vi "populate ring from channel.vi"(7 "instance id":string, 8 "error in":errorcluster, 9 "channel":refnum<class "TBM channel.lvclass">, 10 "ring":refnum<vi>, 11 "engine configuration in":refnum<class "engine configuration.lvclass">) -> (0 "error out":errorcluster, 2 "mapped":bool, 3 "engine configuration out":refnum<class "engine configuration.lvclass">)   [LabVIEW 2013, in "configuration tests.lvlib" / "TEST EDITOR.lvclass"]
uses:
  TEST EDITOR.lvclass
  <vilib>/NI/Tag Bus Module Framework/channel/TBM channel.lvclass
  <vilib>/NI/Module Execution Interface/Engine Configuration/engine configuration.lvclass
  <vilib>/NI/Tag Bus/tag/tag descriptor.lvclass/tag descriptor.ctl
  <vilib>/NI/Tag Bus/tag/tag descriptor.lvclass
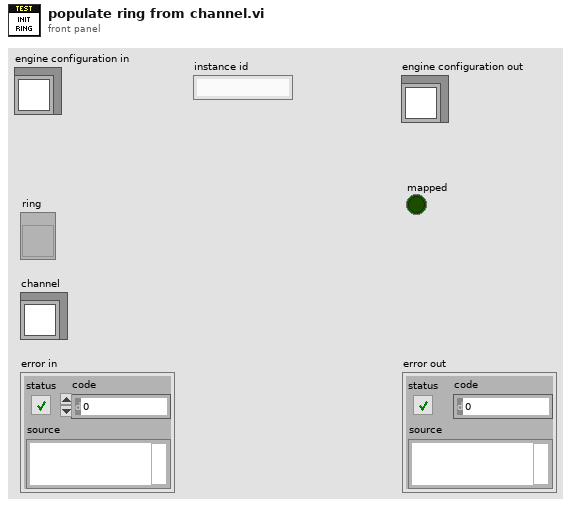
[diagram p1: front panel]
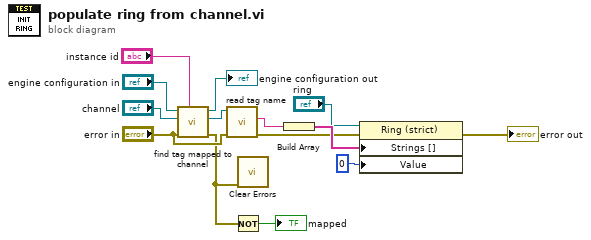
[diagram p0: block diagram]
diagram:
  n1 = call <vilib>:"find tag mapped to channel.vi"("owner"="instance id", "error in"="error in", "channel"="channel", "engine configuration in"="engine configuration in") -> ("error out"=w2:errorcluster, "tag"=w10:refnum<class "tag descriptor.lvclass">, "engine configuration out"=→"engine configuration out":refnum<class "engine configuration.lvclass">)  [unwired: 5 in]
  n2 = call <vilib>:"read tag name.vi"("error in"="error in", "system tag in"=w10) -> ("error out"=w11:errorcluster, "name"=w12:string)  [unwired: 7 in, 1 out]
  n3 = Not(x=w2) -> (.not. x?=→"mapped":bool)
  n4 = call <vilib>:"Clear Errors.vi"("error in (no error)"=w2) -> ()  [unwired: 6 in, 1 out]
  n5 = Build Array(w12) -> (w13:string[])
  n6 = property class="Ring (strict)"(reference="ring", error in=w11, "Strings []"=w13, "Value"=u16 0) -> (error out=→"error out":errorcluster)  [unwired: 1 out]
